vi "Add User Attribute.vi"(0 "iUser Configuration Manager in":refnum<class "iUser Configuration Manager.lvclass">, 5 "Username":string, 7 "Attribute Name":string, 9 "Attribute Value":variant, 11 "error in (no error)":errorcluster) -> (4 "iUser Configuration Manager out":refnum<class "iUser Configuration Manager.lvclass">, 8 "Replaced":bool, 15 "error out":errorcluster)   [LabVIEW 2020, in "User Configuration Manager.lvlib" / "iUser Configuration Manager.lvclass"]
doc: "Adds an attribute to the user."
uses:
  <vilib>/gpm_packages/@cs/user-manager/Source/iUser Configuration Manager/iUser Configuration Manager.lvclass
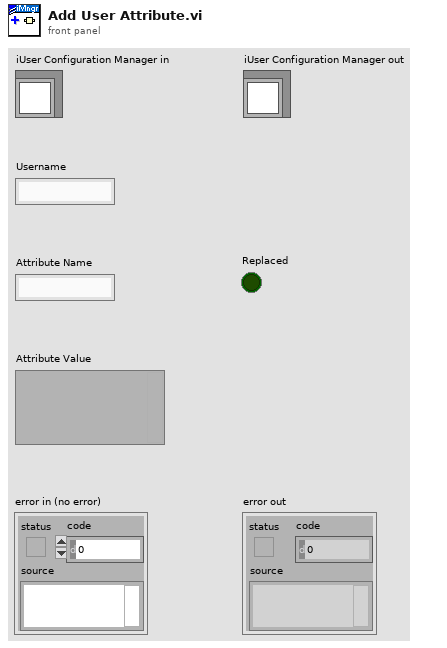
[diagram p1: front panel]
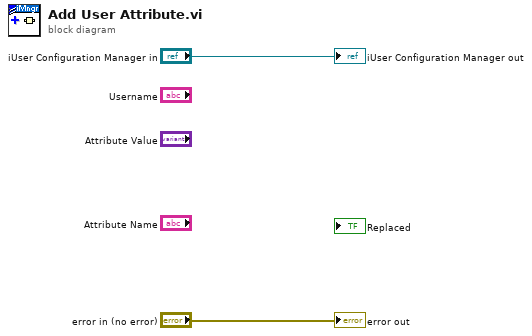
[diagram p0: block diagram]
diagram:
  "error out" <- "error in (no error)"
  "iUser Configuration Manager out" <- "iUser Configuration Manager in"
